vi "Example2.vi"   [LabVIEW 2016]
uses:
  <vilib>/NXT/Dual Mode Library/Waits/Wait_EV3_Color_Color.vi
  <vilib>/NXT/Subs/ColorSensorColors.ctl
  <vilib>/NXT/Block Support/NXT_InputPort.ctl
  <vilib>/NXT/Hardware/Plugins/Tetrix DC Motor/TetrixDCMotorAddress.ctl
  <vilib>/NXT/LegoClasses/BrickReference/BrickReference.lvclass
  <vilib>/NXT/Subs/LVHSConnector.ctl
  <vilib>/NXT/NXTIO Xnodes/NXTIONodeSubVIs/TETRIX IO Stop DC Motors.vi
  <vilib>/NXT/NXTIO Xnodes/NXTIOXNode/NXTIO.xnode
  <vilib>/NXT/NXTIO Xnodes/AddressXNode/NXTIOAddress.xnode
  Test.lvrbt
  <vilib>/NXT/Hardware/Plugins/Tetrix 180 deg Servo/Tetrix180ServoAddress.ctl
  <vilib>/NXT/NXTIO Xnodes/NXTIONodeSubVIs/TETRIX IO Move Servos.vi
  <vilib>/NXT/Dual Mode Library/Waits/Wait_Num.vi
  <vilib>/NXT/NXTIO Xnodes/NXTIONodeSubVIs/TETRIX IO Move DC Motors.vi
types:
  T1 = typedef "NXT_InputPort.ctl" = u32
  T2 = typedef "ColorSensorColors.ctl" = enum16{"No Color", "Black", "Blue", "Green", "Yellow", "Red", "White", "Brown"}
  T3 = typedef "TetrixDCMotorAddress.ctl" = i32
  T4 = typedef "LVHSConnector.ctl" = refnum<class "BrickReference.lvclass">
  T5 = typedef "Tetrix180ServoAddress.ctl" = i32
  T6 = cluster{"Tetrix180Servo":T5, "Tetrix180Servo":T5}
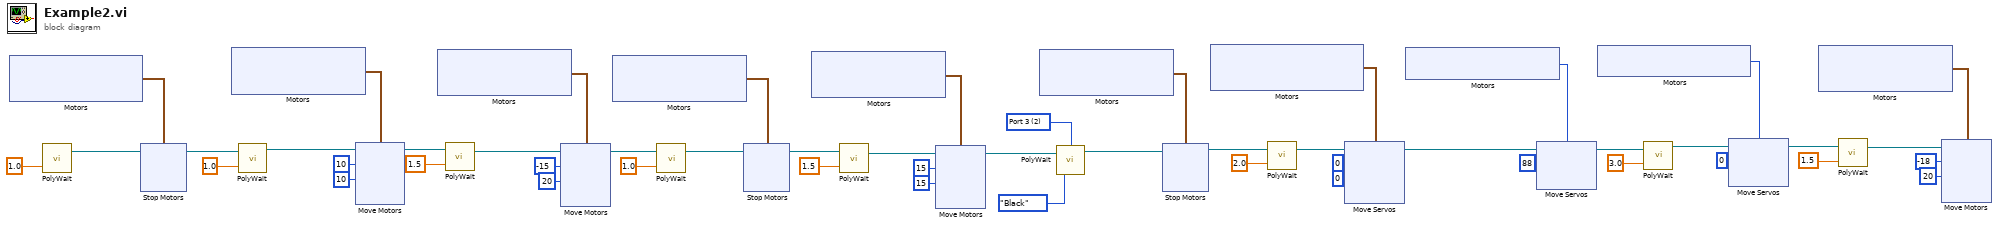
[diagram p0: block diagram]
diagram:
  w50 = T1 2 items=["Port 1", "Port 2", "Port 3", "Port 4"] ("Port (Port 1)")
  n1 = xnode "Motors"() -> ("Motor"=w26:cluster{"TetrixDCMotor":T3, "TetrixDCMotor":T3})
  n2 = call-poly <vilib>:"PolyWait.vi"("Time (1 sec)"=sgl 1.0) -> (2:"NXT/EV3"=w27:T4, 4:"NXT/EV3"=w25:T4)  [unwired: 2 in]
  n3 = xnode "Stop Motors"("Motors"=w26, "NXT/EV3"=w25) -> ("NXT/EV3"=w23:T4)
  n4 = xnode "Motors"() -> ("Motor"=w20:cluster{"TetrixDCMotor":T3, "TetrixDCMotor":T3})
  n5 = call-poly <vilib>:"PolyWait.vi"("Time (1 sec)"=sgl 1.0, "NXT/EV3"=w23) -> ("NXT/EV3"=w19:T4)  [unwired: 2 in]
  n6 = xnode "Move Motors"("Power/Speed 2"=i8 10, "Power/Speed 1"=i8 10, "Motors"=w20, "NXT/EV3"=w19) -> ("NXT/EV3"=w17:T4)
  n7 = xnode "Motors"() -> ("Motor"=w16:cluster{"TetrixDCMotor":T3, "TetrixDCMotor":T3})
  n8 = call-poly <vilib>:"PolyWait.vi"("Time (1 sec)"=sgl 1.5, "NXT/EV3"=w17) -> ("NXT/EV3"=w13:T4)  [unwired: 2 in]
  n9 = xnode "Move Motors"("Power/Speed 2"=i8 20, "Power/Speed 1"=i8 -15, "Motors"=w16, "NXT/EV3"=w13) -> ("NXT/EV3"=w11:T4)
  n10 = xnode "Motors"() -> ("Motor"=w10:cluster{"TetrixDCMotor":T3, "TetrixDCMotor":T3})
  n11 = call-poly <vilib>:"PolyWait.vi"("Time (1 sec)"=sgl 1.0, "NXT/EV3"=w11) -> ("NXT/EV3"=w9:T4)  [unwired: 2 in]
  n12 = xnode "Stop Motors"("Motors"=w10, "NXT/EV3"=w9) -> ("NXT/EV3"=w7:T4)
  n13 = xnode "Motors"() -> ("Motor"=w4:cluster{"TetrixDCMotor":T3, "TetrixDCMotor":T3})
  n14 = call-poly <vilib>:"PolyWait.vi"("Time (1 sec)"=sgl 1.5, "NXT/EV3"=w7) -> ("NXT/EV3"=w3:T4)  [unwired: 2 in]
  n15 = xnode "Move Motors"("Power/Speed 2"=i8 15, "Power/Speed 1"=i8 15, "Motors"=w4, "NXT/EV3"=w3) -> ("NXT/EV3"=w2:T4)
  n16 = xnode "Motors"() -> ("Motor"=w48:cluster{"TetrixDCMotor":T3, "TetrixDCMotor":T3})
  n17 = call-poly <vilib>:"PolyWait.vi"("Color (Red)"=ColorSensorColors."Black", "NXT/EV3"=w2, "Port (Port 1)"=w50) -> ("NXT/EV3"=w49:T4)  [unwired: 1 in]
  n18 = xnode "Stop Motors"("Motors"=w48, "NXT/EV3"=w49) -> ("NXT/EV3"=w30:T4)
  n19 = xnode "Motors"() -> ("Motor"=w47:T6)
  n20 = call-poly <vilib>:"PolyWait.vi"("Time (1 sec)"=sgl 2.0, "NXT/EV3"=w30) -> ("NXT/EV3"=w1:T4)  [unwired: 2 in]
  n21 = xnode "Move Servos"("Position 2"=u8 0, "Position 1"=u8 0, "Motors"=w47, "NXT/EV3"=w1) -> ("NXT/EV3"=w44:T4)
  n22 = xnode "Motors"() -> ("Motor"=w43:T5)
  n23 = xnode "Move Servos"("Position 1"=u8 88, "Motors"=w43, "NXT/EV3"=w44) -> ("NXT/EV3"=w40:T4)
  n24 = xnode "Motors"() -> ("Motor"=w38:T5)
  n25 = call-poly <vilib>:"PolyWait.vi"("Time (1 sec)"=sgl 3.0, "NXT/EV3"=w40) -> ("NXT/EV3"=w37:T4)  [unwired: 2 in]
  n26 = xnode "Move Servos"("Position 1"=u8 0, "Motors"=w38, "NXT/EV3"=w37) -> ("NXT/EV3"=w35:T4)
  n27 = xnode "Motors"() -> ("Motor"=w32:cluster{"TetrixDCMotor":T3, "TetrixDCMotor":T3})
  n28 = call-poly <vilib>:"PolyWait.vi"("Time (1 sec)"=sgl 1.5, "NXT/EV3"=w35) -> ("NXT/EV3"=w31:T4)  [unwired: 2 in]
  n29 = xnode "Move Motors"("Power/Speed 2"=i8 20, "Power/Speed 1"=i8 -18, "Motors"=w32, "NXT/EV3"=w31) -> ()  [unwired: 1 out]
